vi "CAN_Init.vi"(8 "error in (no error)":errorcluster caption="错误输入（无错误）", 10 "VCI_INIT_CONFIG":T2={"AccCode"=0, "AccMask"=4294967295, "Reserved"=0, "Filter"=1, "Timing0"=9, "Timing1"=28, "Mode"=0} {"Timing1" format="%x"; "Timing0" format="%x"; "Filter" format="%x"; "AccMask" format="%x"}, 11 "General_Input":T1={"DevType"=1, "DevIndex"=0, "CANIndex"=0} {"CANIndex" items=["0", "1"]; "DevType" items=["PCI5121"=1, "PCI9810"=2, "USBCAN1"=3, "USBCAN2"=4, "PCI9820"=5, "CAN232"=6, "PCI5110"=7, "CANLite(mini)"=8, "ISA9620"=9, "ISA5420"=10, "PC104CAN"=11, "CANETE"=12, "DNP9810"=13, "PCI9840B"=14, "PC104C2"=15, "PCI9820I"=16]}) -> (0 "错误输出":errorcluster, 2 "return":u32, 3 "General_Output":T1={"DevType"=1, "DevIndex"=0, "CANIndex"=0} {"CANIndex" items=["0", "1"]; "DevType" items=["PCI5121"=1, "PCI9810"=2, "USBCAN1"=3, "USBCAN2"=4, "PCI9820"=5, "CAN232"=6, "PCI5110"=7, "CANLite(mini)"=8, "ISA9620"=9, "ISA5420"=10, "PC104CAN"=11, "CANETE"=12, "DNP9810"=13, "PCI9840B"=14, "PC104C2"=15, "PCI9820I"=16]})   [LabVIEW 2012]
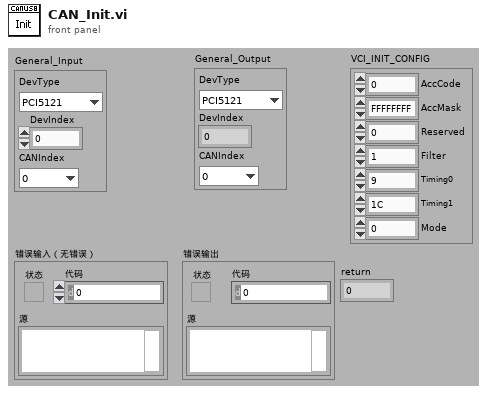
[diagram p1: front panel]
types:
  T1 = cluster{"DevType":u16, "DevIndex":u32, "CANIndex":u16}
  T2 = cluster{"AccCode":u32, "AccMask":u32, "Reserved":u32, "Filter":u8, "Timing0":u8, "Timing1":u8, "Mode":u8}
  T3 = cluster{"DevType":u32, "DevIndex":u32, "CANIndex":u32}
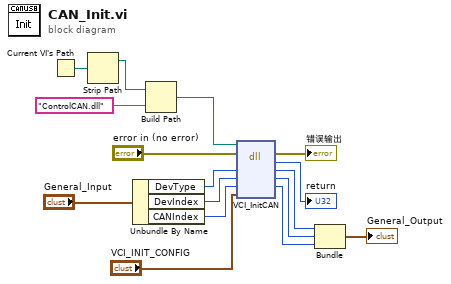
[diagram p0: block diagram]
diagram:
  n1 = Current VI's Path() -> (path=w7:path)
  n2 = Strip Path(path=w7) -> (stripped path=w8:path)  [unwired: 1 out]
  n3 = Unbundle By Name("General_Input") -> ("DevType"=w12:u16, "DevIndex"=w11:u32, "CANIndex"=w10:u16)
  n4 = Build Path(base path=w8, name or relative path="ControlCAN.dll" ("名称或相对路径")) -> (appended path=w6:path)
  n5 = dll-call lib="?" fn="VCI_InitCAN"(path in=w6, error in="error in (no error)", "DevType"=w12, "DevIndex"=w11, "CANIndex"=w10, "pInitConfig"="VCI_INIT_CONFIG") -> (error out=→"错误输出":errorcluster, "return"=→"return":u32, "DevType"=w1:u32, "DevIndex"=w4:u32, "CANIndex"=w3:u32)  [unwired: 2 in, 1 out]
  n6 = Bundle("DevType"=w1, "DevIndex"=w4, "CANIndex"=w3) -> (→"General_Output":T3)  [unwired: 1 in]
